vi "Write DataElements.vi"(8 "error in (no error)":errorcluster, 10 "Data elements":refnum<class "DatagridElement.lvclass">[][](array[class]), 11 "D_Datagrid in":refnum<class "D_Datagrid.lvclass">) -> (0 "error out":errorcluster, 3 "D_Datagrid out":refnum<class "D_Datagrid.lvclass">)   [LabVIEW 2018, in "D Datagrid Library.lvlib" / "D_Datagrid.lvclass"]
uses:
  D_Datagrid.lvclass
  DatagridElement/DatagridElement.lvclass
  D_Datagrid.lvclass/D_Datagrid.ctl
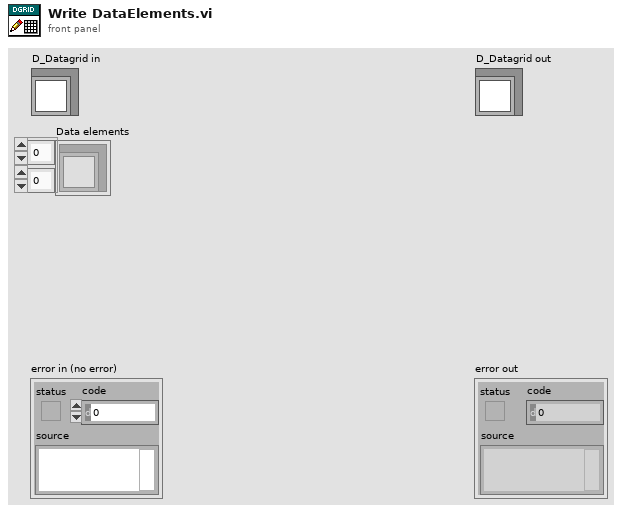
[diagram p1: front panel]
types:
  T1 = typedef "D Datagrid Library.lvlib/D_Datagrid.lvclass/State Data.ctl" = cluster{"Data elements":refnum<class "DatagridElement.lvclass">[][], "Auto-update indicator":bool}
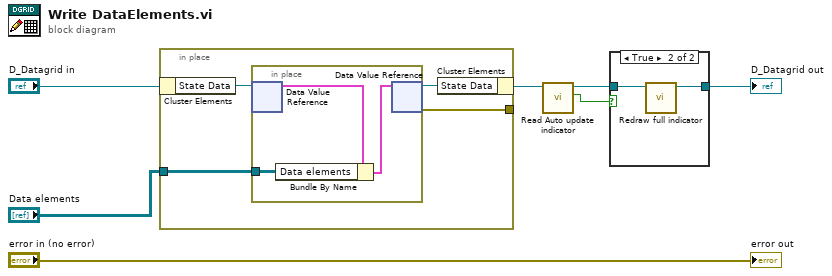
[diagram p0: block diagram]
diagram:
  n1 = in-place {
    in-place-border: "Data elements" -> [w10]
    in-place-border: [w8] -> _
    n2 = in-place-cluster #1("D_Datagrid in") -> ("State Data"=w11:refnum<data-value>)
    n3 = in-place {
      in-place-border: w10 -> [w14]
      n4 = in-place-dvr #2(w11) -> (w13:T1)  [unwired: 1 out]
      n5 = Bundle By Name(cluster=w13, "Data elements"=w14) -> (w12:T1)
      n6 = in-place-dvr #2(w12) -> (w9:refnum<data-value>, w8:errorcluster)
    }
    n7 = in-place-cluster #1("State Data"=w9) -> (w4:refnum<class "D_Datagrid.lvclass">)
  }
  n8 = call "Read Auto update indicator.vi"("D_Datagrid in"=w4) -> ("Auto-update indicator"=w1:bool, "D_Datagrid out"=w3:refnum<class "D_Datagrid.lvclass">)  [unwired: 8 in, 1 out]
  n9 = case shown="True" w1 {
    tunnel: w3 -> [w15 w17]
    tunnel: [w15 w16] -> w6
    frame False {
    }
    frame True {
      n10 = call "Redraw full indicator.vi"("D_Datagrid in"=w17) -> ("D_Datagrid out"=w16:refnum<class "D_Datagrid.lvclass">)  [unwired: 9 in, 1 out]
    }
  }
  "D_Datagrid out" <- w6
  "error out" <- "error in (no error)"
